vi "Get Next.vi"(0 "Name Space in":refnum<class "Name Space.lvclass">, 1 "Linked List Ref":refnum<data-value>, 5 "Active Unique ID":string, 9 "Active Element Index":i32, 11 "error in (no error)":errorcluster) -> (3 "Linked List Ref out":refnum<data-value>, 4 "Executioner out":refnum<class "Executioner.lvclass">, 6 "Active Unique ID out":string, 8 "Test Executive Ref out":refnum<data-value>, 10 "Active Element Index out":i32, 12 "Found":bool, 13 "Complete":bool, 14 "Stop":bool, 15 "error out":errorcluster)   [LabVIEW 2019, in "Test Executive.lvlib" / "Name Space.lvclass"]
uses:
  <vilib>/gpm_packages/@cs/test-executive/Source/Test Executive/Name Space/Name Space.lvclass
  C:/Program Files/National Instruments/LabVIEW 2019/vi.lib/gpm_packages/@cs/test-executive/Source/Test Executive/Executioner/Executioner.lvclass
  <vilib>/gpm_packages/@cs/test-executive/Source/Test Executive/Executioner/Executioner.lvclass
  <vilib>/gpm_packages/@cs/linked-list/Source/Linked List/ILinkedList/ILinked List.lvclass
  <vilib>/gpm_packages/@cs/test-executive/Source/Test Executive/ITestExecutive/ITest Executive.lvclass
  <vilib>/gpm_packages/@cs/linked-list/Source/Linked List/Linked List Ref/Linked List Ref.lvclass
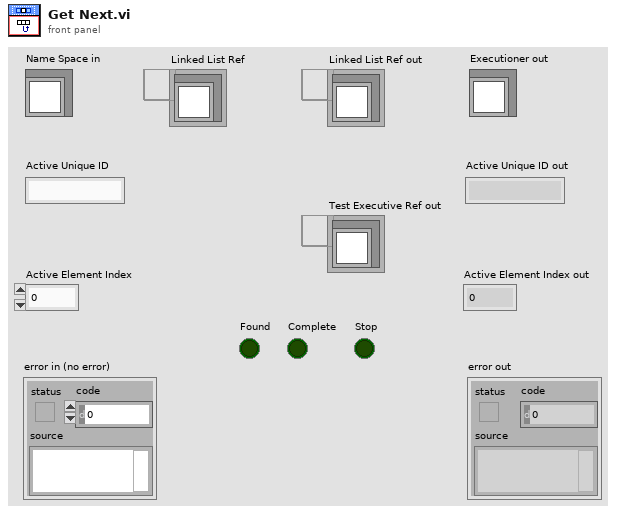
[diagram p1: front panel]
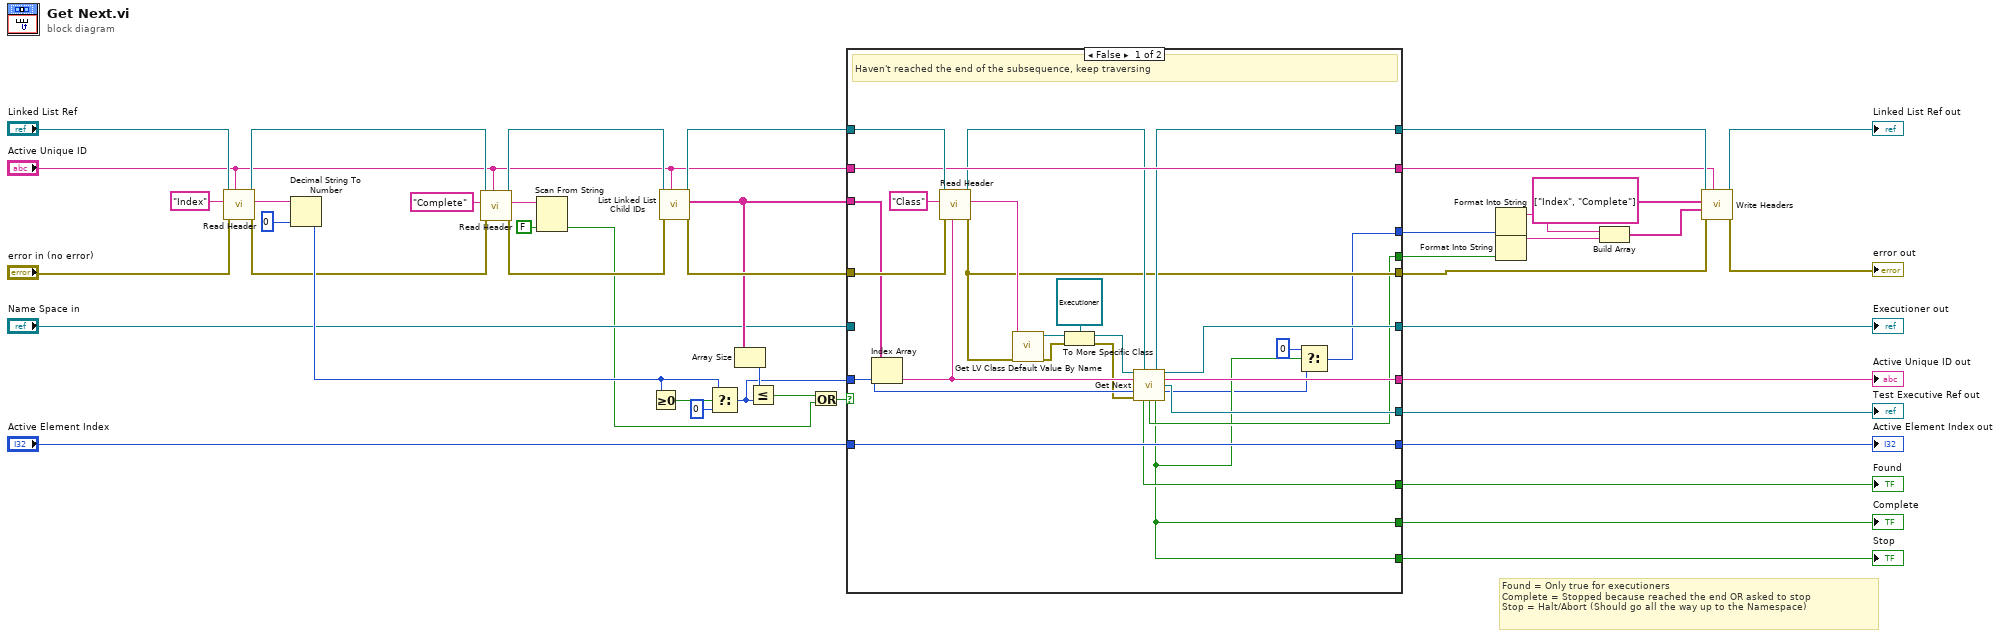
[diagram p0: block diagram]
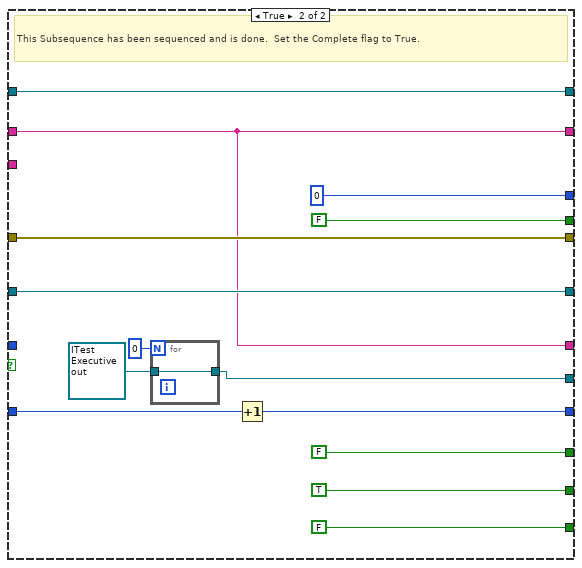
[diagram p2: hidden frame]
diagram:
  # "Found = Only true for executioners\nComplete = Stopped because reached the end OR asked to stop\nStop = Halt/Abort (Should go all the way up to the Namespace)"
  n1 = call <vilib>:"Read Header.vi"("Linked List ID"="Active Unique ID", "error in (no error)"="error in (no error)", "Header Name"="Index" ("Attribute Name"), "Linked List Ref"="Linked List Ref") -> ("error out"=w4:errorcluster, "Header Value"=w17:string, "Linked List Ref out"=w7:refnum<data-value>)  [unwired: 4 in, 1 out]
  n2 = Decimal String To Number(string=w17, default (0L)=0 ("Attribute")) -> (number=w41:i32)  [unwired: 1 in, 1 out]
  n3 = call <vilib>:"Read Header.vi"("Linked List ID"="Active Unique ID", "error in (no error)"=w4, "Header Name"="Complete" ("Attribute Name"), "Linked List Ref"=w7) -> ("error out"=w3:errorcluster, "Header Value"=w9:string, "Linked List Ref out"=w6:refnum<data-value>)  [unwired: 4 in, 1 out]
  n4 = Scan From String(input string=w9, default 1=FALSE) -> (output 1=w2:bool)  [unwired: 3 in, 3 out]
  n5 = Greater Or Equal To 0?(x=w41) -> (x >= 0?=w44:bool)
  n6 = call <vilib>:"List Linked List Child IDs.vi"("Linked List ID"="Active Unique ID", "error in (no error)"=w3, "Linked List Ref"=w6) -> ("error out"=w39:errorcluster, "Child IDs"=w32:string[], "Linked List Ref out"=w40:refnum<data-value>)  [unwired: 6 in]
  n7 = Select(t=w41, s=w44, f=0) -> (s? t:f=w38:i32)
  n8 = Array Size(array=w32) -> (size(s)=w42:i32)
  n9 = Less Or Equal?(x=w42, y=w38) -> (x <= y?=w19:bool)
  n10 = Or(x=w19, y=w2) -> (x .or. y?=w1:bool)
  n11 = case shown="False" w1 {
    tunnel: [w64 w84] -> w37
    tunnel: w40 -> [w70 w84]
    tunnel: [w56 w83] -> w36
    tunnel: w39 -> [w69 w83]
    tunnel: w38 -> [w63 _]
    tunnel: "Active Element Index" -> [w54 w81]
    tunnel: [w67 w76] -> w34
    tunnel: "Active Unique ID" -> [w67 w76]
    tunnel: [w51 w82] -> w23
    tunnel: "Name Space in" -> [_ w82]
    tunnel: [w54 w80] -> w27
    tunnel: [w53 FALSE] -> w26
    tunnel: [w47 TRUE] -> w25
    tunnel: [w47 FALSE] -> w24
    tunnel: [w52 w76] -> w22
    tunnel: [w45 0] -> w35
    tunnel: [w49 FALSE] -> w33
    tunnel: w32 -> [w66 _]
    tunnel: [w50 w71] -> w11
    frame False {
      # "Haven't reached the end of the subsequence, keep traversing"
      n12 = Index Array(array=w66, index=w63) -> (element=w62:string)
      n13 = call <vilib>:"Read Header.vi"("Linked List ID"=w62, "error in (no error)"=w69, "Header Name"="Class", "Linked List Ref"=w70) -> ("error out"=w56:errorcluster, "Header Value"=w61:string, "Linked List Ref out"=w65:refnum<data-value>)  [unwired: 4 in, 1 out]
      n14 = call <vilib>:"Get LV Class Default Value By Name.vi"("error in (no error)"=w56, "class name"=w61) -> ("error out"=w57:errorcluster, "object"=w60:refnum<class>)  [unwired: 8 in]
      n15 = To More Specific Class(target class=refnum<class "Executioner.lvclass"> refnum ("Test Executive.lvlib:Executioner.lvclass"), reference=w60, error in=w57) -> (specific class reference=w55:refnum<class "Executioner.lvclass">, error out=w58:errorcluster)
      n16 = call-dynamic "Get Next.vi"("Executioner in"=w55, "Linked List Ref"=w65, "Active Unique ID"=w62, "Active Element Index"=w63, "error in (no error)"=w58) -> ("Linked List Ref out"=w64:refnum<data-value>, "Executioner out"=w51:refnum<class "Executioner.lvclass">, "Active Unique ID out"=w52:string, "Test Executive Ref out"=w50:refnum<data-value>, "Active Element Index out"=w46:i32, "Found"=w53:bool, "Complete"=w49:bool, "Stop"=w47:bool)  [unwired: 2 in, 1 out]
      n17 = Select(t=0, s=w47, f=w46) -> (s? t:f=w45:i32)
    }
    frame True {
      # "This Subsequence has been sequenced and is done.  Set the Complete flag to True."
      n18 = for {
        N: 0 -> [_]
        tunnel: refnum<data-value> refnum ("Test Executive Ref out") -> [w85]
        tunnel: [w85] -> w71
      }
      n19 = Increment(x=w81) -> (x+1=w80:i32)
    }
  }
  "Executioner out" <- w23
  "Active Unique ID out" <- w22
  "Active Element Index out" <- w27
  "Found" <- w26
  "Complete" <- w25
  "Stop" <- w24
  "Test Executive Ref out" <- w11
  n20 = Format Into String(w35) -> (resulting string=w14:string)  [unwired: 3 in, 1 out]
  n21 = Format Into String(w33) -> (resulting string=w13:string)  [unwired: 3 in, 1 out]
  n22 = Build Array(w14, w13) -> (w12:string[])
  n23 = call <vilib>:"Write Headers.vi"("Linked List ID"=w34, "error in (no error)"=w36, "Header Values"=w12, "Header Names"=string[] ["Index", "Complete"], "Linked List Ref"=w37) -> ("error out"=→"error out":errorcluster, "Linked List Ref out"=→"Linked List Ref out":refnum<data-value>)  [unwired: 5 in]
